vi "Auto Aim.vi"   [LabVIEW 2023]
uses:
  <vilib>/Rock Robotics/Network Tables/NT Read Number.vi
types:
  T1 = cluster{"offsetAngle H":dbl, "offsetAngle V":dbl, "area":dbl, "skew":dbl}
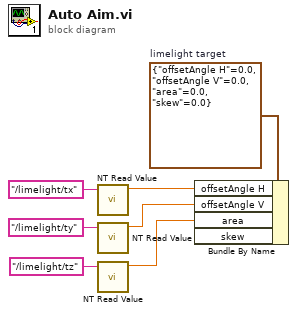
[diagram p0: block diagram]
diagram:
  w4 = T1 {"offsetAngle H"=0.0, "offsetAngle V"=0.0, "area"=0.0, "skew"=0.0}  # limelight target
  n1 = call-poly <vilib>:"NT Read Value.vi"("name"="/limelight/tx" ("Name")) -> ("value"=w3:dbl)  [unwired: 8 in, 2 out]
  n2 = call-poly <vilib>:"NT Read Value.vi"("name"="/limelight/ty" ("Name")) -> ("value"=w2:dbl)  [unwired: 8 in, 2 out]
  n3 = call-poly <vilib>:"NT Read Value.vi"("name"="/limelight/tz" ("Name")) -> ("value"=w1:dbl)  [unwired: 8 in, 2 out]
  n4 = Bundle By Name(cluster=w4, "offsetAngle H"=w3, "offsetAngle V"=w2, "area"=w1) -> ()  [unwired: 1 in, 1 out]
